vi "VirtualTestInstrument.vi"(8 "error in (no error)":errorcluster, 10 "Message":T1={"Command"="", "Data"=variant(string ""), "ID"=""}, 11 "RemoteControl":refnum<class "RemoteControl.lvclass">) -> (0 "error out":errorcluster, 2 "processed Message":T1={"Command"="", "Data"=variant(string ""), "ID"=""}, 3 "RemoteControl":refnum<class "RemoteControl.lvclass">)   [LabVIEW 2019, in "RemoteControl.lvclass"]
uses:
  RemoteControl.lvclass
  Typedefs/Message--Cluster.ctl
  RemoteControl.lvclass/RemoteControl.ctl
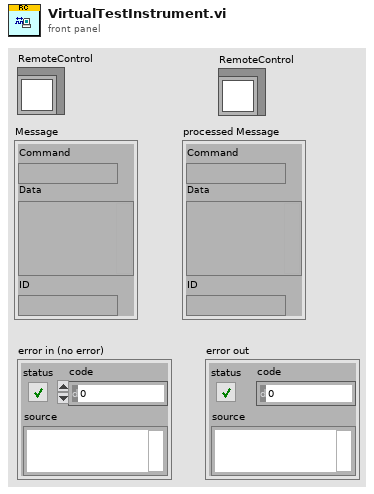
[diagram p1: front panel]
types:
  T1 = typedef "RemoteControl.lvclass/Message--Cluster.ctl" = cluster{"Command":string, "Data":variant, "ID":string}
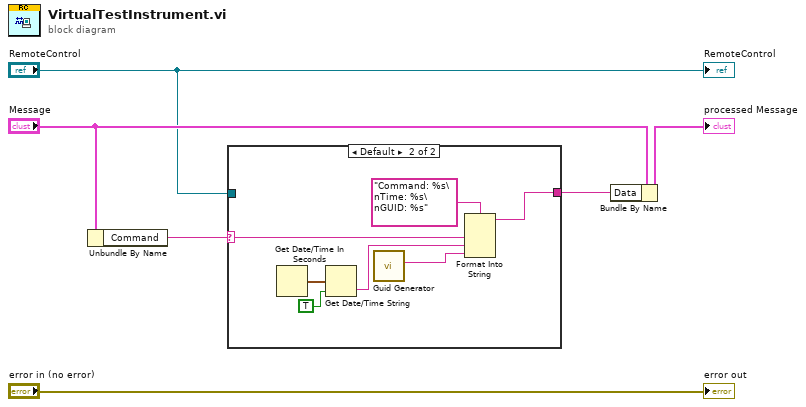
[diagram p0: block diagram]
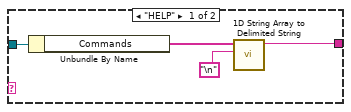
[diagram p2: hidden frame]
diagram:
  n1 = Unbundle By Name("Message") -> ("Command"=w1:string)
  n2 = case shown="Default" w1 {
    selector: w1 -> [_ w12]
    tunnel: [w8 w11] -> w2
    tunnel: "RemoteControl" -> [w10 _]
    frame "HELP" {
      n3 = Unbundle By Name(w10) -> ("Commands"=w9:string[])
      n4 = call <vilib>:"1D String Array to Delimited String.vi"("delimiter"="\n", "string array"=w9) -> ("delimited string"=w8:string)  [unwired: 9 in]
    }
    frame Default {
      n5 = Get Date/Time In Seconds() -> (seconds since 1Jan1904=w16:timestamp)
      n6 = Get Date/Time String(seconds (now)=w16, want seconds? (F)=TRUE) -> (time string=w13:string)  [unwired: 1 in, 1 out]
      n7 = call <vilib>:"Guid Generator.vi"() -> ("GUID"=w14:string)  [unwired: 10 in, 1 out]
      n8 = Format Into String(format string="Command: %s\nTime: %s\nGUID: %s", w12, w13, w14) -> (resulting string=w11:string)  [unwired: 2 in, 1 out]
    }
  }
  n9 = Bundle By Name(cluster="Message", "Data"=w2) -> (→"processed Message":T1)
  "error out" <- "error in (no error)"
  "RemoteControl" <- "RemoteControl"
